vi "Get Parent Class Name.vi"(8 "error in (no error)":errorcluster, 11 "lvclass path":path) -> (0 "error out":errorcluster, 3 "parent class name":string)   [LabVIEW 2021, in "MeasurementService Editor.lvlib"]
uses:
  MeasurementService Editor.lvlib
  <vilib>/xml/NI_XML.lvlib
  <resource>/objmgr/DOMUserDefRef.rc
  <vilib>/xml/Close Reference(Node).vi
  <vilib>/xml/Close Reference(NNMap).vi
  <vilib>/xml/Load XML File.vi
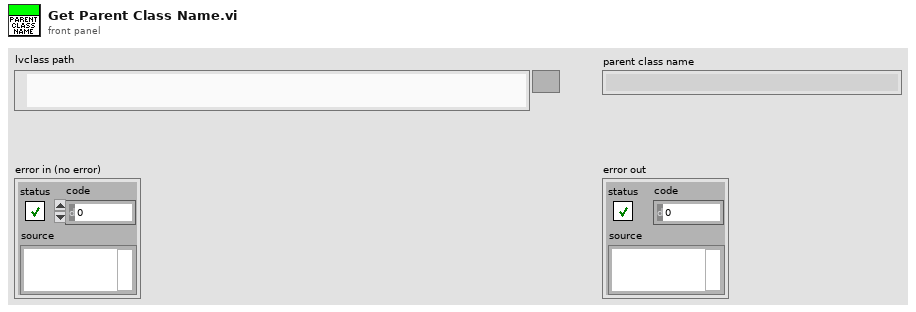
[diagram p1: front panel]
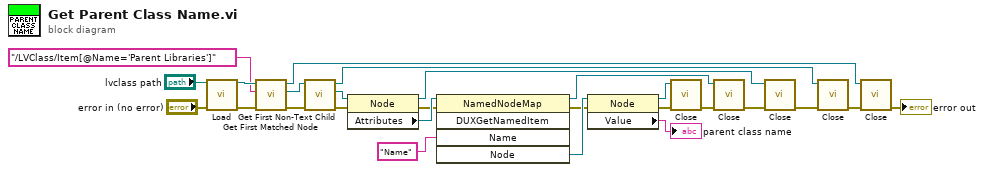
[diagram p0: block diagram]
diagram:
  n1 = call-poly <vilib>:"Load.vi"("path to XML document"="lvclass path", "error in (no error)"="error in (no error)") -> ("DOM document out"=w25:refnum<k20>, "error out"=w24:errorcluster)  [unwired: 11 in, 1 out]
  n2 = call <vilib>:"Get First Matched Node.vi"("error in (no error)"=w24, "XPath expression"="/LVClass/Item[@Name='Parent Libraries']", "node in"=w25) -> ("error out"=w20:errorcluster, "node result"=w21:refnum<k20>, "node out"=w22:refnum<k20>)  [unwired: 6 in]
  n3 = call <vilib>:"Get First Non-Text Child.vi"("error in (no error)"=w20, "node in"=w21) -> ("error out"=w15:errorcluster, "child node"=w19:refnum<k20>, "node out"=w3:refnum<k20>)  [unwired: 6 in, 1 out]
  n4 = property class="Node"(reference=w19, error in=w15) -> (reference out=w6:refnum<k20>, error out=w14:errorcluster, "Attributes"=w18:refnum<k20>)
  n5 = invoke class="NamedNodeMap" method="DUXGetNamedItem"(reference=w18, error in=w14, "Name"="Name") -> (reference out=w7:refnum<k20>, error out=w13:errorcluster, "Node"=w16:refnum<k20>)  [unwired: 2 in, 2 out]
  n6 = property class="Node"(reference=w16, error in=w13) -> (reference out=w8:refnum<k20>, error out=w11:errorcluster, "Value"=→"parent class name":string)
  n7 = call-poly <vilib>:"Close.vi"("error in (no error)"=w11, "node"=w8) -> ("error out"=w10:errorcluster)  [unwired: 7 in]
  n8 = call-poly <vilib>:"Close.vi"("error in (no error)"=w10, "named node map"=w7) -> ("error out"=w9:errorcluster)  [unwired: 7 in]
  n9 = call-poly <vilib>:"Close.vi"("error in (no error)"=w9, "node"=w6) -> ("error out"=w5:errorcluster)  [unwired: 7 in]
  n10 = call-poly <vilib>:"Close.vi"("error in (no error)"=w5, "node"=w3) -> ("error out"=w4:errorcluster)  [unwired: 7 in]
  n11 = call-poly <vilib>:"Close.vi"("error in (no error)"=w4, "node"=w22) -> ("error out"=→"error out":errorcluster)  [unwired: 7 in]
